vi "Generate Waveforms.vi"(1 "Single Tone.lvclass":refnum<class "Single Tone.lvclass">) -> (0 "Waveforms":waveform(dbl)[](array[waveform]))   [LabVIEW 2010, in "Single Tone.lvclass"]
doc: "This method creates a sine wave output based on the Frequency and Duration values that were acquired by Generate Tone.vi."
uses:
  Single Tone.lvclass
  Single Tone.lvclass/Single Tone.ctl
  <vilib>/measure/NI_MABase.lvlib
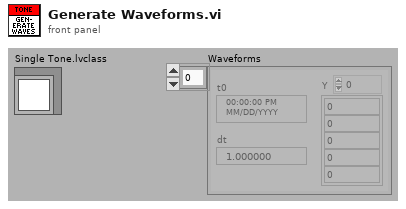
[diagram p1: front panel]
types:
  T1 = cluster{"Samples per Second":dbl, "Number of Samples":dbl}
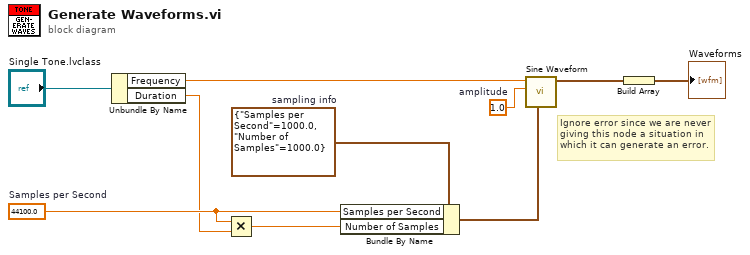
[diagram p0: block diagram]
diagram:
  w6 = 44100.0  # Samples per Second
  w7 = T1 {"Samples per Second"=1000.0, "Number of Samples"=1000.0}  # sampling info
  w8 = 1.0  # amplitude
  # "Ignore error since we are never giving this node a situation in which it can generate an error."
  n1 = Unbundle By Name "Unbundle By Name"("Single Tone.lvclass") -> ("Frequency"=w9:dbl, "Duration"=w5:dbl)
  n2 = Multiply(x=w6, y=w5) -> (x*y=w4:dbl)
  n3 = Bundle By Name "Bundle By Name"(cluster=w7, "Samples per Second"=w6, "Number of Samples"=w4) -> (w3:T1)
  n4 = call <vilib>:"Sine Waveform.vi"("sampling info"=w3, "amplitude"=w8, "frequency"=w9) -> ("signal out"=w2:waveform(dbl))  [unwired: 7 in, 1 out]
  n5 = Build Array "Build Array"(w2) -> (→"Waveforms":waveform(dbl)[])
